vi "ModbusTCP-Demo.vi"() -> ()   [LabVIEW 2013]
uses:
  <userlib>/nimodbus121/86/vi.lib/NI Modbus.llb/MB Ethernet Master Query Read Discrete Inputs (poly).vi
  <userlib>/nimodbus121/86/vi.lib/NI Modbus.llb/MB Ethernet Master Query Read Input Registers (poly).vi
  <userlib>/nimodbus121/86/vi.lib/NI Modbus.llb/MB Ethernet Master Query Write Multiple Coils (poly).vi
  <userlib>/nimodbus121/86/vi.lib/NI Modbus.llb/MB Ethernet Master Query Write Multiple Registers (poly).vi
panel:
  in  "LED0闪烁":bool
  in  "BEEP":bool
  in  "LED1":bool
  in  "LED0":bool
  in  "DAC电压值：":dbl min=0.0 max=3.4 step=0.1 format="%0.1f V"
  out "WK_UP":bool
  out "KEY2":bool
  out "KEY1":bool
  out "KEY0":bool
  out "光敏传感器":u16 format="%d L"
  out "内部温度传感器":dbl format="%0.2f ℃"
  out "电压(PA5-ADC)":dbl format="%0.2f V"
  in  "端口：":u16=502
  in  "ModbusIP：":string="192.168.10.22"
  in  "Stop":bool
  # "正点原子 探索者开发板\nSTM32F407 Modbus TCP 通信测试上位机"
  # "Write Multiple Coils [000]"
  # "Write Multiple Registers [400]"
  # "Read Discrete Inputs [100]"
  # "Read Input Registers [300]"
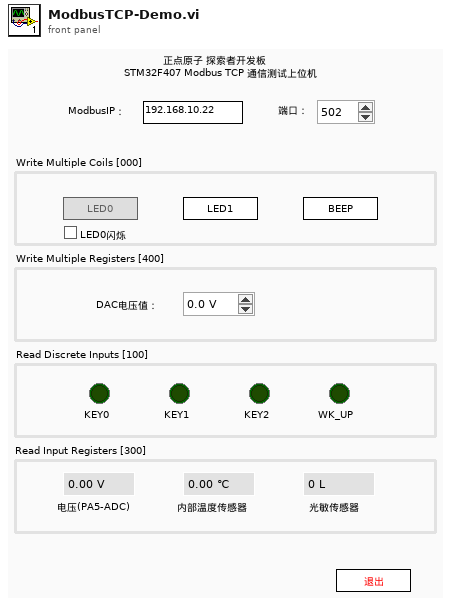
[diagram p1: front panel]
types:
  T1 = enum8{"Enabled", "Disabled", "Disabled and Grayed Out"}
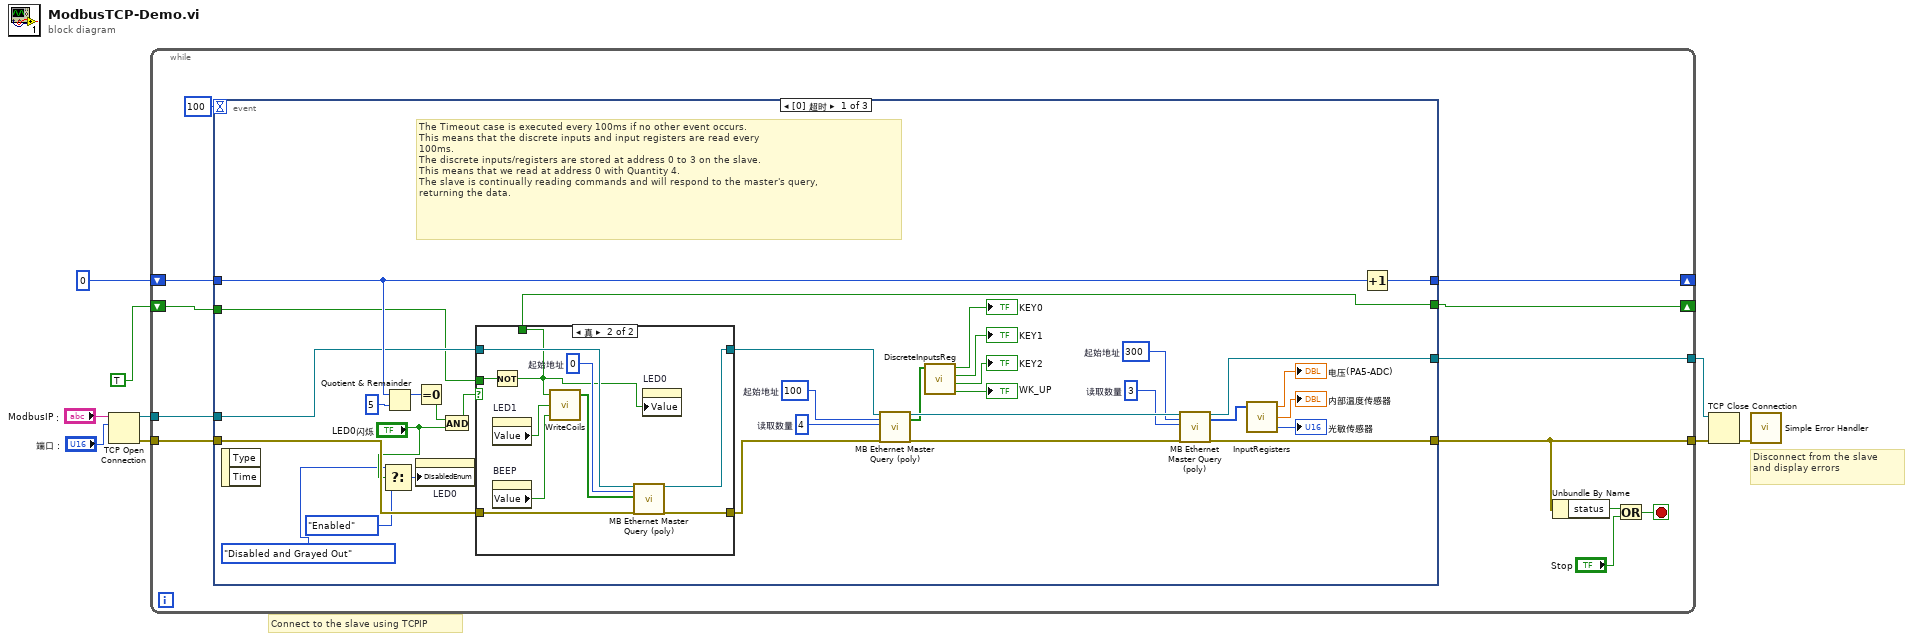
[diagram p0: block diagram]
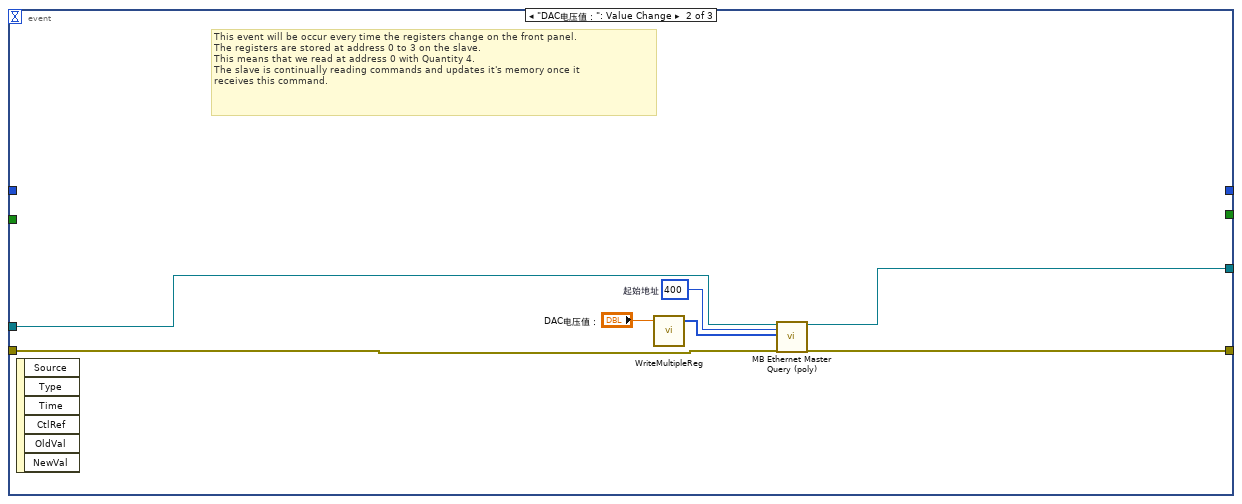
[diagram p3: hidden frame]
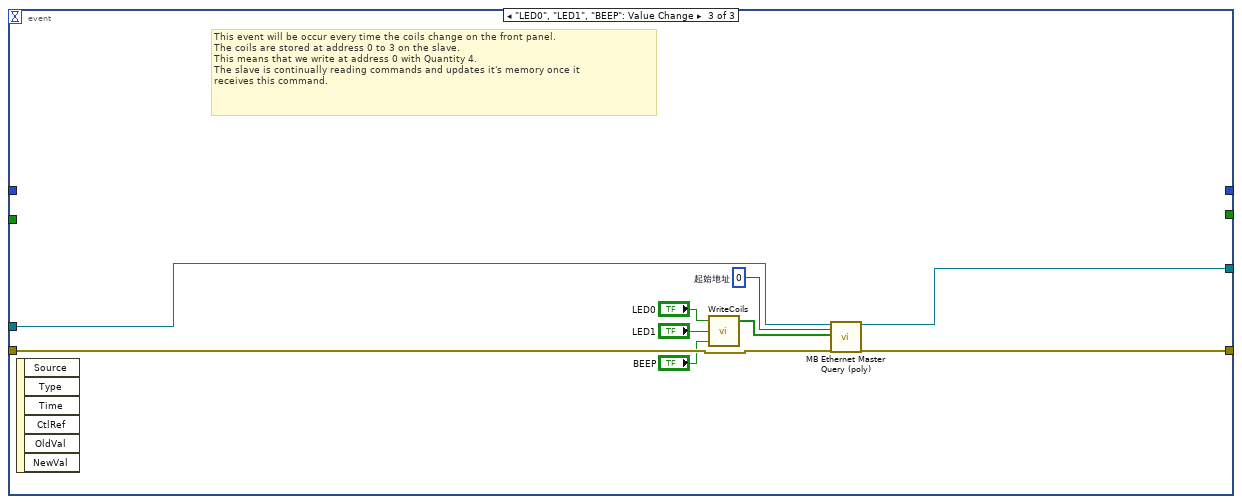
[diagram p4: hidden frame]
diagram:
  # "Disconnect from the slave\nand display errors"
  # "Connect to the slave using TCPIP"
  n1 = TCP Open Connection(address="ModbusIP：", remote port or service name="端口：") -> (connection ID=w7:refnum<k5>, error out=w6:errorcluster)  [unwired: 1 in, 2 out]
  n2 = while {
    tunnel: [w18] -> w4
    tunnel: w7 -> [w16]
    tunnel: w6 -> [w15]
    tunnel: [w14] -> w3
    shift-right: [w12] -> _
    shift-left: 0 -> [w13]
    shift-right: [w10] -> _
    shift-left: TRUE -> [w11]
    stop <- w21 stop-if-true
    n3 = event shown="[0] 超时" {
      selector: _ -> [_ _ _]
      dyn-events: _ -> [_ _ _]
      timeout: 100 -> [_ _ _]
      tunnel: [w47 w71 w83] -> w18
      tunnel: w16 -> [w33 w74 w82]
      tunnel: w15 -> [w32 w73 w80]
      tunnel: [w48 w70 w79] -> w14
      tunnel: w13 -> [w34 _ _]
      tunnel: [w37 _ _] -> w12
      tunnel: w11 -> [w29 _ _]
      tunnel: [w28 _ _] -> w10
      event Timeout {
        w49 = u16 3  # 读取数量
        w50 = u16 300  # 起始地址
        w53 = u16 4  # 读取数量
        w54 = u16 100  # 起始地址
        # "The Timeout case is executed every 100ms if no other event occurs.\nThis means that the discrete inputs and input registers are read every \n100ms.\nThe discrete inputs/registers are stored at address 0 to 3 on the slave.\nThis means that we read at address 0 with Quantity 4.\nThe slave is continually reading commands and will respond to the master's query,\nreturning the data."
        n4 = event-data() -> ()  [unwired: 3 out]
        n5 = Select(t=T1."Disabled and Grayed Out" ("禁用"), s="LED0闪烁", f=T1."Enabled" ("禁用")) -> (s? t:f=w22:T1)
        n6 = Quotient & Remainder(x=w34, y=5) -> (x-y*floor(x/y)=w35:i32)  [unwired: 1 out]
        n7 = Equal To 0?(x=w35) -> (x = 0?=w27:bool)
        n8 = property on="LED0" class="Bool (严格)"("DisabledEnum"=w22) -> ()  [unwired: 2 in, 2 out]
        n9 = And(x=w27, y="LED0闪烁") -> (x .and. y?=w26:bool)
        n10 = case shown="真" w26 {
          tunnel: w33 -> [w57 w65]
          tunnel: w32 -> [w56 w64]
          tunnel: [w57 w63] -> w31
          tunnel: [w56 w62] -> w30
          tunnel: w29 -> [w55 w59]
          tunnel: [w55 w58] -> w28
          frame False {
          }
          frame True {
            w66 = u16 0  # 起始地址
            n11 = Not(x=w59) -> (.not. x?=w58:bool)
            n12 = property on="LED1" class="Bool (严格)"() -> ("Value"=w61:bool)  [unwired: 2 in, 2 out]
            n13 = property on="BEEP" class="Bool (严格)"() -> ("Value"=w60:bool)  [unwired: 2 in, 2 out]
            n14 = call "WriteCoils.vi"("BEEP"=w60, "LED1"=w61, "LED0"=w58) -> ("Coils to Write Ouput"=w67:bool[])  [unwired: 2 in]
            n15 = call-poly <userlib>:"MB Ethernet Master Query (poly).vi"("TCP Connection Refnum in"=w65, "Starting Address"=w66, "Coils"=w67, "error in"=w64) -> ("TCP Connection Refnum (dup)"=w63:refnum<k5>, "error out"=w62:errorcluster)  [unwired: 3 in, 11 out]
            n16 = property on="LED0" class="Bool (严格)"("Value"=w58) -> ()  [unwired: 2 in, 2 out]
          }
        }
        n17 = call-poly <userlib>:"MB Ethernet Master Query (poly).vi"("TCP Connection Refnum in"=w31, "Starting Address"=w54, "Quantity"=w53, "error in"=w30) -> ("TCP Connection Refnum (dup)"=w52:refnum<k5>, "Discrete Inputs"=w42:bool[], "error out"=w51:errorcluster)  [unwired: 1 in, 12 out]
        n18 = call "DiscreteInputsReg.vi"("Discrete Inputs"=w42) -> ("WK_UP"=→"WK_UP":bool, "KEY2"=→"KEY2":bool, "KEY1"=→"KEY1":bool, "KEY0"=→"KEY0":bool)  [unwired: 3 in]
        n19 = call-poly <userlib>:"MB Ethernet Master Query (poly).vi"("TCP Connection Refnum in"=w52, "Starting Address"=w50, "Quantity"=w49, "error in"=w51) -> ("TCP Connection Refnum (dup)"=w48:refnum<k5>, "Input Registers"=w46:u16[], "error out"=w47:errorcluster)  [unwired: 1 in, 12 out]
        n20 = call "InputRegisters.vi"("Input Registers"=w46) -> ("光敏传感器"=→"光敏传感器":u16, "内部温度传感器"=→"内部温度传感器":dbl, "电压(PA5-ADC)"=→"电压(PA5-ADC)":dbl)  [unwired: 2 in]
        n21 = Increment(x=w34) -> (x+1=w37:i32)
      }
      event "DAC电压值：": Value Change {
        w72 = u16 400  # 起始地址
        # "This event will be occur every time the registers change on the front panel.\nThe registers are stored at address 0 to 3 on the slave.\nThis means that we read at address 0 with Quantity 4.\nThe slave is continually reading commands and updates it's memory once it\nreceives this command."
        n22 = event-data() -> ()  [unwired: 7 out]
        n23 = call "WriteMultipleReg.vi"("DAC电压值"="DAC电压值：") -> ("数组"=w68:u16[])  [unwired: 4 in]
        n24 = call-poly <userlib>:"MB Ethernet Master Query (poly).vi"("TCP Connection Refnum in"=w74, "Starting Address"=w72, "Registers"=w68, "error in"=w73) -> ("TCP Connection Refnum (dup)"=w70:refnum<k5>, "error out"=w71:errorcluster)  [unwired: 3 in, 11 out]
      }
      event "LED0", "LED1", "BEEP": Value Change {
        w81 = u16 0  # 起始地址
        # "This event will be occur every time the coils change on the front panel.\nThe coils are stored at address 0 to 3 on the slave.\nThis means that we write at address 0 with Quantity 4.\nThe slave is continually reading commands and updates it's memory once it\nreceives this command."
        n25 = event-data() -> ()  [unwired: 7 out]
        n26 = call "WriteCoils.vi"("BEEP"="BEEP", "LED1"="LED1", "LED0"="LED0") -> ("Coils to Write Ouput"=w78:bool[])  [unwired: 2 in]
        n27 = call-poly <userlib>:"MB Ethernet Master Query (poly).vi"("TCP Connection Refnum in"=w82, "Starting Address"=w81, "Coils"=w78, "error in"=w80) -> ("TCP Connection Refnum (dup)"=w79:refnum<k5>, "error out"=w83:errorcluster)  [unwired: 3 in, 11 out]
      }
    }
    n28 = Unbundle By Name(w18) -> ("status"=w19:bool)
    n29 = Or(x=w19, y="Stop") -> (x .or. y?=w21:bool)
  }
  n30 = TCP Close Connection(connection ID=w3, error in (no error)=w4) -> (error out=w5:errorcluster)  [unwired: 2 out]
  n31 = call <vilib>:"Simple Error Handler.vi"("error in (no error)"=w5) -> ()  [unwired: 1 in, 8 out]
